vi "Get Electrical Angle.vi"(7 "timeout (1s)":dbl=1.0 min=0.0, 8 "error in (no error)":errorcluster, 11 "SDO object in":refnum<k20>) -> (0 "error out":errorcluster, 1 "completion code":u32 format="%.0x", 2 "I32 data":i16, 3 "SDO object out":refnum<k20>)   [LabVIEW 2016]
uses:
  <vilib>/CANopenLib/CANOPEN.llb/CANopen SDO Read [I16].vi
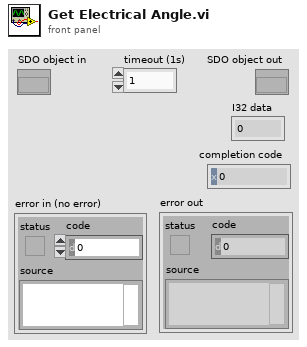
[diagram p1: front panel]
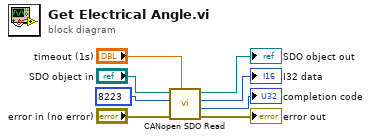
[diagram p0: block diagram]
diagram:
  n1 = call-poly <vilib>:"CANopen SDO Read.vi"("timeout (1s)"="timeout (1s)", "error in (no error)"="error in (no error)", "object index"=u16 8223, "SDO object in"="SDO object in") -> ("error out"=→"error out":errorcluster, "completion code"=→"completion code":u32, "I16 data"=→"I32 data":i16, "SDO object out"=→"SDO object out":refnum<k20>)  [unwired: 4 in]
